vi "_EnumEditor_SetActualStrings.vi"(8 "error in (no error)":errorcluster, 10 "ActualStrings":string[](array[string]), 11 "_EnumEditor in":refnum<class "_EnumEditor.lvclass">) -> (0 "error out":errorcluster, 3 "_EnumEditor out":refnum<class "_EnumEditor.lvclass">)   [LabVIEW 2014, in "_EnumEditor.lvclass"]
uses:
  _EnumEditor.lvclass
  _EnumEditor.lvclass/_EnumEditor.ctl
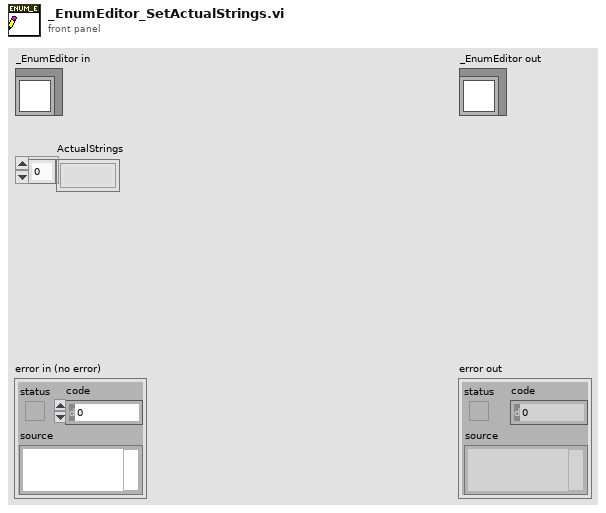
[diagram p1: front panel]
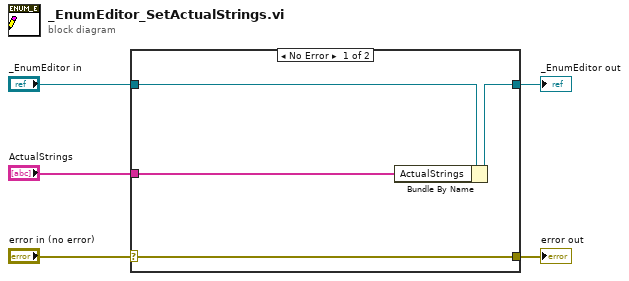
[diagram p0: block diagram]
diagram:
  n1 = case shown="No Error" "error in (no error)" {
    selector: "error in (no error)" -> [w9 w10]
    tunnel: [w9 w10] -> w4
    tunnel: [w7 w11] -> w2
    tunnel: "_EnumEditor in" -> [w8 w11]
    tunnel: "ActualStrings" -> [w6 _]
    frame No Error {
      n2 = Bundle By Name(cluster=w8, "ActualStrings"=w6) -> (w7:refnum<class "_EnumEditor.lvclass">)
    }
    frame Error {
    }
  }
  "error out" <- w4
  "_EnumEditor out" <- w2
